vi "main(Test DQMH modules).vi"() -> ()   [LabVIEW 2018, in "Application.lvlib"] (continued)
            n1625 = Select(t="Quece timeout", s=w3888, f=w3885) -> (s? t:f=w3884:string)
            n1626 = call "string log (SubVI).vi"("Enum"=enum16{"Init", "Log", "Read"}."Log", "state Name"=w3884) -> ()  [unwired: 8 in, 2 out]
          }
          frame condition #1 {
          }
        }
        n1627 = call "progress string(SubVI).vi"("String 3"=w3850, "String in"=w3851) -> ("String out"=w3852:string)  [unwired: 9 in]
        n1628 = call "FGV Driver Data.vi"("DUT index(1-60)"=w3849) -> ("DUT SC"=w3848:bool)  [unwired: 7 in, 3 out]
        n1629 = case shown="False" w3848 {
          tunnel: [w3877 _] -> w3857
          tunnel: w3854 -> [w3876 _]
          frame False {
            w3864 = T11 {"command"="", "command data"=variant} ("element")
            w3863 = "MEAS.mux6_1"
            n1630 = To Variant(anything=T4."mux6-1_channel0" ("mux6_1(3wires)_encode")) -> (Variant=w3862:variant)
            n1631 = To Variant(anything=T4."mux6_1_channel1_3" ("mux6_1(3wires)_encode")) -> (Variant=w3874:variant)
            n1632 = To Variant(anything=T4."mux6-1_channel1_2" ("mux6_1(3wires)_encode")) -> (Variant=w3872:variant)
            n1633 = Bundle By Name(cluster=w3864, "command"=w3863, "command data"=w3872) -> (w3871:T11)
            n1634 = Bundle By Name(cluster=w3864, "command"=w3863, "command data"=w3874) -> (w3870:T11)
            n1635 = Bundle By Name(cluster=w3864, "command"=w3863, "command data"=w3862) -> ()  [unwired: 1 out]
            n1636 = Bundle By Name(cluster=w3864, "command"="MEAS.DMM dual read") -> (w3868:T11)
            n1637 = Build Array(w3871, w3870, w3868) -> (w3866:T11[])
            n1638 = Reverse 1D Array(array=w3866) -> (reversed array=w3867:T11[])
            n1639 = for {
              tunnel: [w3883] -> w3877 mode=indexing
              tunnel: w3876 -> [w3882]
              tunnel: w3867 -> [w3881] mode=indexing
              n1640 = Unbundle By Name(w3881) -> ("command"=w3880:string, "command data"=w3879:variant)
              n1641 = call "App enquece.vi"("Priority Enquece"=TRUE, "command data"=w3879, "command"=w3880, "queue in"=w3882) -> ("error out"=w3883:errorcluster)  [unwired: 6 in, 1 out]
            }
          }
          frame True {
          }
        }
        n1642 = Merge Errors(w3855, w3857) -> (w3856:errorcluster)
      }
      frame "Test DRV 8" {
        w3890 = 8  # DUT index(0-59)
        n1643 = disable-structure shown="LOGGING==TRUE" {
          disable-tunnel: w3891 -> [w3926 _]
          frame condition #0 (active) {
            n1644 = Empty String/Path?(string/path=w3926) -> (empty?=w3929:bool)
            n1645 = Select(t="Quece timeout", s=w3929, f=w3926) -> (s? t:f=w3925:string)
            n1646 = call "string log (SubVI).vi"("Enum"=enum16{"Init", "Log", "Read"}."Log", "state Name"=w3925) -> ()  [unwired: 8 in, 2 out]
          }
          frame condition #1 {
          }
        }
        n1647 = call "progress string(SubVI).vi"("String 3"=w3891, "String in"=w3892) -> ("String out"=w3893:string)  [unwired: 9 in]
        n1648 = call "FGV Driver Data.vi"("DUT index(1-60)"=w3890) -> ("DUT SC"=w3889:bool)  [unwired: 7 in, 3 out]
        n1649 = case shown="False" w3889 {
          tunnel: [w3918 _] -> w3898
          tunnel: w3895 -> [w3917 _]
          frame False {
            w3905 = T11 {"command"="", "command data"=variant} ("element")
            w3904 = "MEAS.mux6_1"
            n1650 = To Variant(anything=T4."mux6-1_channel0" ("mux6_1(3wires)_encode")) -> (Variant=w3903:variant)
            n1651 = To Variant(anything=T4."mux6_1_channel2_3" ("mux6_1(3wires)_encode")) -> (Variant=w3915:variant)
            n1652 = To Variant(anything=T4."mux6_1_channel2_2" ("mux6_1(3wires)_encode")) -> (Variant=w3913:variant)
            n1653 = Bundle By Name(cluster=w3905, "command"=w3904, "command data"=w3913) -> (w3912:T11)
            n1654 = Bundle By Name(cluster=w3905, "command"=w3904, "command data"=w3915) -> (w3911:T11)
            n1655 = Bundle By Name(cluster=w3905, "command"=w3904, "command data"=w3903) -> ()  [unwired: 1 out]
            n1656 = Bundle By Name(cluster=w3905, "command"="MEAS.DMM dual read") -> (w3909:T11)
            n1657 = Build Array(w3912, w3911, w3909) -> (w3907:T11[])
            n1658 = Reverse 1D Array(array=w3907) -> (reversed array=w3908:T11[])
            n1659 = for {
              tunnel: [w3924] -> w3918 mode=indexing
              tunnel: w3917 -> [w3923]
              tunnel: w3908 -> [w3922] mode=indexing
              n1660 = Unbundle By Name(w3922) -> ("command"=w3921:string, "command data"=w3920:variant)
              n1661 = call "App enquece.vi"("Priority Enquece"=TRUE, "command data"=w3920, "command"=w3921, "queue in"=w3923) -> ("error out"=w3924:errorcluster)  [unwired: 6 in, 1 out]
            }
          }
          frame True {
          }
        }
        n1662 = Merge Errors(w3896, w3898) -> (w3897:errorcluster)
      }
      frame "Test DRV 9" {
        w3931 = 9  # DUT index(0-59)
        n1663 = disable-structure shown="LOGGING==TRUE" {
          disable-tunnel: w3932 -> [w3967 _]
          frame condition #0 (active) {
            n1664 = Empty String/Path?(string/path=w3967) -> (empty?=w3970:bool)
            n1665 = Select(t="Quece timeout", s=w3970, f=w3967) -> (s? t:f=w3966:string)
            n1666 = call "string log (SubVI).vi"("Enum"=enum16{"Init", "Log", "Read"}."Log", "state Name"=w3966) -> ()  [unwired: 8 in, 2 out]
          }
          frame condition #1 {
          }
        }
        n1667 = call "progress string(SubVI).vi"("String 3"=w3932, "String in"=w3933) -> ("String out"=w3934:string)  [unwired: 9 in]
        n1668 = call "FGV Driver Data.vi"("DUT index(1-60)"=w3931) -> ("DUT SC"=w3930:bool)  [unwired: 7 in, 3 out]
        n1669 = case shown="False" w3930 {
          tunnel: [w3959 _] -> w3939
          tunnel: w3936 -> [w3958 _]
          frame False {
            w3946 = T11 {"command"="", "command data"=variant} ("element")
            w3945 = "MEAS.mux6_1"
            n1670 = To Variant(anything=T4."mux6-1_channel0" ("mux6_1(3wires)_encode")) -> (Variant=w3944:variant)
            n1671 = To Variant(anything=T4."mux6_1_channel3_3" ("mux6_1(3wires)_encode")) -> (Variant=w3956:variant)
            n1672 = To Variant(anything=T4."mux6_1_channel3_2" ("mux6_1(3wires)_encode")) -> (Variant=w3954:variant)
            n1673 = Bundle By Name(cluster=w3946, "command"=w3945, "command data"=w3954) -> (w3953:T11)
            n1674 = Bundle By Name(cluster=w3946, "command"=w3945, "command data"=w3956) -> (w3952:T11)
            n1675 = Bundle By Name(cluster=w3946, "command"=w3945, "command data"=w3944) -> ()  [unwired: 1 out]
            n1676 = Bundle By Name(cluster=w3946, "command"="MEAS.DMM dual read") -> (w3950:T11)
            n1677 = Build Array(w3953, w3952, w3950) -> (w3948:T11[])
            n1678 = Reverse 1D Array(array=w3948) -> (reversed array=w3949:T11[])
            n1679 = for {
              tunnel: [w3965] -> w3959 mode=indexing
              tunnel: w3958 -> [w3964]
              tunnel: w3949 -> [w3963] mode=indexing
              n1680 = Unbundle By Name(w3963) -> ("command"=w3962:string, "command data"=w3961:variant)
              n1681 = call "App enquece.vi"("Priority Enquece"=TRUE, "command data"=w3961, "command"=w3962, "queue in"=w3964) -> ("error out"=w3965:errorcluster)  [unwired: 6 in, 1 out]
            }
          }
          frame True {
          }
        }
        n1682 = Merge Errors(w3937, w3939) -> (w3938:errorcluster)
      }
      frame "Test DRV 10" {
        w3972 = 10  # DUT index(0-59)
        n1683 = disable-structure shown="LOGGING==TRUE" {
          disable-tunnel: w3973 -> [w4008 _]
          frame condition #0 (active) {
            n1684 = Empty String/Path?(string/path=w4008) -> (empty?=w4011:bool)
            n1685 = Select(t="Quece timeout", s=w4011, f=w4008) -> (s? t:f=w4007:string)
            n1686 = call "string log (SubVI).vi"("Enum"=enum16{"Init", "Log", "Read"}."Log", "state Name"=w4007) -> ()  [unwired: 8 in, 2 out]
          }
          frame condition #1 {
          }
        }
        n1687 = call "progress string(SubVI).vi"("String 3"=w3973, "String in"=w3974) -> ("String out"=w3975:string)  [unwired: 9 in]
        n1688 = call "FGV Driver Data.vi"("DUT index(1-60)"=w3972) -> ("DUT SC"=w3971:bool)  [unwired: 7 in, 3 out]
        n1689 = case shown="False" w3971 {
          tunnel: [w4000 _] -> w3980
          tunnel: w3977 -> [w3999 _]
          frame False {
            w3987 = T11 {"command"="", "command data"=variant} ("element")
            w3986 = "MEAS.mux6_1"
            n1690 = To Variant(anything=T4."mux6-1_channel0" ("mux6_1(3wires)_encode")) -> (Variant=w3985:variant)
            n1691 = To Variant(anything=T4."mux6_1_channel4_3" ("mux6_1(3wires)_encode")) -> (Variant=w3997:variant)
            n1692 = To Variant(anything=T4."mux6_1_channel4_2" ("mux6_1(3wires)_encode")) -> (Variant=w3995:variant)
            n1693 = Bundle By Name(cluster=w3987, "command"=w3986, "command data"=w3995) -> (w3994:T11)
            n1694 = Bundle By Name(cluster=w3987, "command"=w3986, "command data"=w3997) -> (w3993:T11)
            n1695 = Bundle By Name(cluster=w3987, "command"=w3986, "command data"=w3985) -> ()  [unwired: 1 out]
            n1696 = Bundle By Name(cluster=w3987, "command"="MEAS.DMM dual read") -> (w3991:T11)
            n1697 = Build Array(w3994, w3993, w3991) -> (w3989:T11[])
            n1698 = Reverse 1D Array(array=w3989) -> (reversed array=w3990:T11[])
            n1699 = for {
              tunnel: [w4006] -> w4000 mode=indexing
              tunnel: w3999 -> [w4005]
              tunnel: w3990 -> [w4004] mode=indexing
              n1700 = Unbundle By Name(w4004) -> ("command"=w4003:string, "command data"=w4002:variant)
              n1701 = call "App enquece.vi"("Priority Enquece"=TRUE, "command data"=w4002, "command"=w4003, "queue in"=w4005) -> ("error out"=w4006:errorcluster)  [unwired: 6 in, 1 out]
            }
          }
          frame True {
          }
        }
        n1702 = Merge Errors(w3978, w3980) -> (w3979:errorcluster)
      }
      frame "Test DRV 11" {
        w4013 = 11  # DUT index(0-59)
        n1703 = disable-structure shown="LOGGING==TRUE" {
          disable-tunnel: w4014 -> [w4049 _]
          frame condition #0 (active) {
            n1704 = Empty String/Path?(string/path=w4049) -> (empty?=w4052:bool)
            n1705 = Select(t="Quece timeout", s=w4052, f=w4049) -> (s? t:f=w4048:string)
            n1706 = call "string log (SubVI).vi"("Enum"=enum16{"Init", "Log", "Read"}."Log", "state Name"=w4048) -> ()  [unwired: 8 in, 2 out]
          }
          frame condition #1 {
          }
        }
        n1707 = call "progress string(SubVI).vi"("String 3"=w4014, "String in"=w4015) -> ("String out"=w4016:string)  [unwired: 9 in]
        n1708 = call "FGV Driver Data.vi"("DUT index(1-60)"=w4013) -> ("DUT SC"=w4012:bool)  [unwired: 7 in, 3 out]
        n1709 = case shown="False" w4012 {
          tunnel: [w4041 _] -> w4021
          tunnel: w4018 -> [w4040 _]
          frame False {
            w4026 = T11 {"command"="", "command data"=variant} ("element")
            w4028 = "MEAS.mux6_1"
            n1710 = To Variant(anything=T4."mux6-1_channel0" ("mux6_1(3wires)_encode")) -> (Variant=w4027:variant)
            n1711 = To Variant(anything=T4."mux6_1_channel5_3" ("mux6_1(3wires)_encode")) -> (Variant=w4038:variant)
            n1712 = To Variant(anything=T4."mux6_1_channel5_2" ("mux6_1(3wires)_encode")) -> (Variant=w4036:variant)
            n1713 = Bundle By Name(cluster=w4026, "command"=w4028, "command data"=w4036) -> (w4035:T11)
            n1714 = Bundle By Name(cluster=w4026, "command"=w4028, "command data"=w4038) -> (w4034:T11)
            n1715 = Bundle By Name(cluster=w4026, "command"=w4028, "command data"=w4027) -> ()  [unwired: 1 out]
            n1716 = Bundle By Name(cluster=w4026, "command"="MEAS.DMM dual read") -> (w4032:T11)
            n1717 = Build Array(w4035, w4034, w4032) -> (w4030:T11[])
            n1718 = Reverse 1D Array(array=w4030) -> (reversed array=w4031:T11[])
            n1719 = for {
              tunnel: [w4047] -> w4041 mode=indexing
              tunnel: w4040 -> [w4046]
              tunnel: w4031 -> [w4045] mode=indexing
              n1720 = Unbundle By Name(w4045) -> ("command"=w4044:string, "command data"=w4043:variant)
              n1721 = call "App enquece.vi"("Priority Enquece"=TRUE, "command data"=w4043, "command"=w4044, "queue in"=w4046) -> ("error out"=w4047:errorcluster)  [unwired: 6 in, 1 out]
            }
          }
          frame True {
          }
        }
        n1722 = Merge Errors(w4019, w4021) -> (w4020:errorcluster)
      }
      frame "Test DRV 12" {
        w4054 = 12  # DUT index(0-59)
        n1723 = disable-structure shown="LOGGING==TRUE" {
          disable-tunnel: w4055 -> [w4090 _]
          frame condition #0 (active) {
            n1724 = Empty String/Path?(string/path=w4090) -> (empty?=w4093:bool)
            n1725 = Select(t="Quece timeout", s=w4093, f=w4090) -> (s? t:f=w4089:string)
            n1726 = call "string log (SubVI).vi"("Enum"=enum16{"Init", "Log", "Read"}."Log", "state Name"=w4089) -> ()  [unwired: 8 in, 2 out]
          }
          frame condition #1 {
          }
        }
        n1727 = call "progress string(SubVI).vi"("String 3"=w4055, "String in"=w4056) -> ("String out"=w4057:string)  [unwired: 9 in]
        n1728 = call "FGV Driver Data.vi"("DUT index(1-60)"=w4054) -> ("DUT SC"=w4053:bool)  [unwired: 7 in, 3 out]
        n1729 = case shown="False" w4053 {
          tunnel: [w4082 _] -> w4062
          tunnel: w4059 -> [w4081 _]
          frame False {
            w4069 = T11 {"command"="", "command data"=variant} ("element")
            w4068 = "MEAS.mux6_1"
            n1730 = To Variant(anything=T4."mux6-1_channel0" ("mux6_1(3wires)_encode")) -> (Variant=w4067:variant)
            n1731 = To Variant(anything=T4."mux6_1_channel6_3" ("mux6_1(3wires)_encode")) -> (Variant=w4079:variant)
            n1732 = To Variant(anything=T4."mux6_1_channel6_2" ("mux6_1(3wires)_encode")) -> (Variant=w4077:variant)
            n1733 = Bundle By Name(cluster=w4069, "command"=w4068, "command data"=w4077) -> (w4076:T11)
            n1734 = Bundle By Name(cluster=w4069, "command"=w4068, "command data"=w4079) -> (w4075:T11)
            n1735 = Bundle By Name(cluster=w4069, "command"=w4068, "command data"=w4067) -> ()  [unwired: 1 out]
            n1736 = Bundle By Name(cluster=w4069, "command"="MEAS.DMM dual read") -> (w4073:T11)
            n1737 = Build Array(w4076, w4075, w4073) -> (w4071:T11[])
            n1738 = Reverse 1D Array(array=w4071) -> (reversed array=w4072:T11[])
            n1739 = for {
              tunnel: [w4088] -> w4082 mode=indexing
              tunnel: w4081 -> [w4087]
              tunnel: w4072 -> [w4086] mode=indexing
              n1740 = Unbundle By Name(w4086) -> ("command"=w4085:string, "command data"=w4084:variant)
              n1741 = call "App enquece.vi"("Priority Enquece"=TRUE, "command data"=w4084, "command"=w4085, "queue in"=w4087) -> ("error out"=w4088:errorcluster)  [unwired: 6 in, 1 out]
            }
          }
          frame True {
          }
        }
        n1742 = Merge Errors(w4060, w4062) -> (w4061:errorcluster)
      }
      frame "Test DRV 13" {
        w4095 = 13  # DUT index(0-59)
        n1743 = disable-structure shown="LOGGING==TRUE" {
          disable-tunnel: w4096 -> [w4131 _]
          frame condition #0 (active) {
            n1744 = Empty String/Path?(string/path=w4131) -> (empty?=w4134:bool)
            n1745 = Select(t="Quece timeout", s=w4134, f=w4131) -> (s? t:f=w4130:string)
            n1746 = call "string log (SubVI).vi"("Enum"=enum16{"Init", "Log", "Read"}."Log", "state Name"=w4130) -> ()  [unwired: 8 in, 2 out]
          }
          frame condition #1 {
          }
        }
        n1747 = call "progress string(SubVI).vi"("String 3"=w4096, "String in"=w4097) -> ("String out"=w4098:string)  [unwired: 9 in]
        n1748 = call "FGV Driver Data.vi"("DUT index(1-60)"=w4095) -> ("DUT SC"=w4094:bool)  [unwired: 7 in, 3 out]
        n1749 = case shown="False" w4094 {
          tunnel: [w4123 _] -> w4103
          tunnel: w4100 -> [w4122 _]
          frame False {
            w4110 = T11 {"command"="", "command data"=variant} ("element")
            w4109 = "MEAS.mux6_1"
            n1750 = To Variant(anything=T4."mux6-1_channel0" ("mux6_1(3wires)_encode")) -> (Variant=w4108:variant)
            n1751 = To Variant(anything=T4."mux6_1_channel1_3" ("mux6_1(3wires)_encode")) -> (Variant=w4120:variant)
            n1752 = To Variant(anything=T4."mux6-1_channel1_2" ("mux6_1(3wires)_encode")) -> (Variant=w4118:variant)
            n1753 = Bundle By Name(cluster=w4110, "command"=w4109, "command data"=w4118) -> (w4117:T11)
            n1754 = Bundle By Name(cluster=w4110, "command"=w4109, "command data"=w4120) -> (w4116:T11)
            n1755 = Bundle By Name(cluster=w4110, "command"=w4109, "command data"=w4108) -> ()  [unwired: 1 out]
            n1756 = Bundle By Name(cluster=w4110, "command"="MEAS.DMM dual read") -> (w4114:T11)
            n1757 = Build Array(w4117, w4116, w4114) -> (w4112:T11[])
            n1758 = Reverse 1D Array(array=w4112) -> (reversed array=w4113:T11[])
            n1759 = for {
              tunnel: [w4129] -> w4123 mode=indexing
              tunnel: w4122 -> [w4128]
              tunnel: w4113 -> [w4127] mode=indexing
              n1760 = Unbundle By Name(w4127) -> ("command"=w4126:string, "command data"=w4125:variant)
              n1761 = call "App enquece.vi"("Priority Enquece"=TRUE, "command data"=w4125, "command"=w4126, "queue in"=w4128) -> ("error out"=w4129:errorcluster)  [unwired: 6 in, 1 out]
            }
          }
          frame True {
          }
        }
        n1762 = Merge Errors(w4101, w4103) -> (w4102:errorcluster)
      }
      frame "Test DRV 14" {
        w4136 = 14  # DUT index(0-59)
        n1763 = disable-structure shown="LOGGING==TRUE" {
          disable-tunnel: w4137 -> [w4172 _]
          frame condition #0 (active) {
            n1764 = Empty String/Path?(string/path=w4172) -> (empty?=w4175:bool)
            n1765 = Select(t="Quece timeout", s=w4175, f=w4172) -> (s? t:f=w4171:string)
            n1766 = call "string log (SubVI).vi"("Enum"=enum16{"Init", "Log", "Read"}."Log", "state Name"=w4171) -> ()  [unwired: 8 in, 2 out]
          }
          frame condition #1 {
          }
        }
        n1767 = call "progress string(SubVI).vi"("String 3"=w4137, "String in"=w4138) -> ("String out"=w4139:string)  [unwired: 9 in]
        n1768 = call "FGV Driver Data.vi"("DUT index(1-60)"=w4136) -> ("DUT SC"=w4135:bool)  [unwired: 7 in, 3 out]
        n1769 = case shown="False" w4135 {
          tunnel: [w4164 _] -> w4144
          tunnel: w4141 -> [w4163 _]
          frame False {
            w4151 = T11 {"command"="", "command data"=variant} ("element")
            w4150 = "MEAS.mux6_1"
            n1770 = To Variant(anything=T4."mux6_1_channel2_3" ("mux6_1(3wires)_encode")) -> (Variant=w4161:variant)
            n1771 = To Variant(anything=T4."mux6-1_channel0" ("mux6_1(3wires)_encode")) -> (Variant=w4149:variant)
            n1772 = To Variant(anything=T4."mux6_1_channel2_2" ("mux6_1(3wires)_encode")) -> (Variant=w4159:variant)
            n1773 = Bundle By Name(cluster=w4151, "command"=w4150, "command data"=w4159) -> (w4158:T11)
            n1774 = Bundle By Name(cluster=w4151, "command"=w4150, "command data"=w4161) -> (w4157:T11)
            n1775 = Bundle By Name(cluster=w4151, "command"=w4150, "command data"=w4149) -> ()  [unwired: 1 out]
            n1776 = Bundle By Name(cluster=w4151, "command"="MEAS.DMM dual read") -> (w4155:T11)
            n1777 = Build Array(w4158, w4157, w4155) -> (w4153:T11[])
            n1778 = Reverse 1D Array(array=w4153) -> (reversed array=w4154:T11[])
            n1779 = for {
              tunnel: [w4170] -> w4164 mode=indexing
              tunnel: w4163 -> [w4169]
              tunnel: w4154 -> [w4168] mode=indexing
              n1780 = Unbundle By Name(w4168) -> ("command"=w4167:string, "command data"=w4166:variant)
              n1781 = call "App enquece.vi"("Priority Enquece"=TRUE, "command data"=w4166, "command"=w4167, "queue in"=w4169) -> ("error out"=w4170:errorcluster)  [unwired: 6 in, 1 out]
            }
          }
          frame True {
          }
        }
        n1782 = Merge Errors(w4142, w4144) -> (w4143:errorcluster)
      }
      frame "Test DRV 15" {
        w4177 = 15  # DUT index(0-59)
        n1783 = disable-structure shown="LOGGING==TRUE" {
          disable-tunnel: w4178 -> [w4213 _]
          frame condition #0 (active) {
            n1784 = Empty String/Path?(string/path=w4213) -> (empty?=w4216:bool)
            n1785 = Select(t="Quece timeout", s=w4216, f=w4213) -> (s? t:f=w4212:string)
            n1786 = call "string log (SubVI).vi"("Enum"=enum16{"Init", "Log", "Read"}."Log", "state Name"=w4212) -> ()  [unwired: 8 in, 2 out]
          }
          frame condition #1 {
          }
        }
        n1787 = call "progress string(SubVI).vi"("String 3"=w4178, "String in"=w4179) -> ("String out"=w4180:string)  [unwired: 9 in]
        n1788 = call "FGV Driver Data.vi"("DUT index(1-60)"=w4177) -> ("DUT SC"=w4176:bool)  [unwired: 7 in, 3 out]
        n1789 = case shown="False" w4176 {
          tunnel: [w4205 _] -> w4185
          tunnel: w4182 -> [w4204 _]
          frame False {
            w4192 = T11 {"command"="", "command data"=variant} ("element")
            w4191 = "MEAS.mux6_1"
            n1790 = To Variant(anything=T4."mux6-1_channel0" ("mux6_1(3wires)_encode")) -> (Variant=w4190:variant)
            n1791 = To Variant(anything=T4."mux6_1_channel3_3" ("mux6_1(3wires)_encode")) -> (Variant=w4202:variant)
            n1792 = To Variant(anything=T4."mux6_1_channel3_2" ("mux6_1(3wires)_encode")) -> (Variant=w4200:variant)
            n1793 = Bundle By Name(cluster=w4192, "command"=w4191, "command data"=w4200) -> (w4199:T11)
            n1794 = Bundle By Name(cluster=w4192, "command"=w4191, "command data"=w4202) -> (w4198:T11)
            n1795 = Bundle By Name(cluster=w4192, "command"=w4191, "command data"=w4190) -> ()  [unwired: 1 out]
            n1796 = Bundle By Name(cluster=w4192, "command"="MEAS.DMM dual read") -> (w4196:T11)
            n1797 = Build Array(w4199, w4198, w4196) -> (w4194:T11[])
            n1798 = Reverse 1D Array(array=w4194) -> (reversed array=w4195:T11[])
            n1799 = for {
              tunnel: [w4211] -> w4205 mode=indexing
              tunnel: w4204 -> [w4210]
              tunnel: w4195 -> [w4209] mode=indexing
              n1800 = Unbundle By Name(w4209) -> ("command"=w4208:string, "command data"=w4207:variant)
              n1801 = call "App enquece.vi"("Priority Enquece"=TRUE, "command data"=w4207, "command"=w4208, "queue in"=w4210) -> ("error out"=w4211:errorcluster)  [unwired: 6 in, 1 out]
            }
          }
          frame True {
          }
        }
        n1802 = Merge Errors(w4183, w4185) -> (w4184:errorcluster)
      }
      frame "Test DRV 16" {
        w4218 = 16  # DUT index(0-59)
        n1803 = disable-structure shown="LOGGING==TRUE" {
          disable-tunnel: w4219 -> [w4254 _]
          frame condition #0 (active) {
            n1804 = Empty String/Path?(string/path=w4254) -> (empty?=w4257:bool)
            n1805 = Select(t="Quece timeout", s=w4257, f=w4254) -> (s? t:f=w4253:string)
            n1806 = call "string log (SubVI).vi"("Enum"=enum16{"Init", "Log", "Read"}."Log", "state Name"=w4253) -> ()  [unwired: 8 in, 2 out]
          }
          frame condition #1 {
          }
        }
        n1807 = call "progress string(SubVI).vi"("String 3"=w4219, "String in"=w4220) -> ("String out"=w4221:string)  [unwired: 9 in]
        n1808 = call "FGV Driver Data.vi"("DUT index(1-60)"=w4218) -> ("DUT SC"=w4217:bool)  [unwired: 7 in, 3 out]
        n1809 = case shown="False" w4217 {
          tunnel: [w4246 _] -> w4226
          tunnel: w4223 -> [w4245 _]
          frame False {
            w4233 = T11 {"command"="", "command data"=variant} ("element")
            w4232 = "MEAS.mux6_1"
            n1810 = To Variant(anything=T4."mux6-1_channel0" ("mux6_1(3wires)_encode")) -> (Variant=w4231:variant)
            n1811 = To Variant(anything=T4."mux6_1_channel4_3" ("mux6_1(3wires)_encode")) -> (Variant=w4243:variant)
            n1812 = To Variant(anything=T4."mux6_1_channel4_2" ("mux6_1(3wires)_encode")) -> (Variant=w4241:variant)
            n1813 = Bundle By Name(cluster=w4233, "command"=w4232, "command data"=w4241) -> (w4240:T11)
            n1814 = Bundle By Name(cluster=w4233, "command"=w4232, "command data"=w4243) -> (w4239:T11)
            n1815 = Bundle By Name(cluster=w4233, "command"=w4232, "command data"=w4231) -> ()  [unwired: 1 out]
            n1816 = Bundle By Name(cluster=w4233, "command"="MEAS.DMM dual read") -> (w4237:T11)
            n1817 = Build Array(w4240, w4239, w4237) -> (w4235:T11[])
            n1818 = Reverse 1D Array(array=w4235) -> (reversed array=w4236:T11[])
            n1819 = for {
              tunnel: [w4252] -> w4246 mode=indexing
              tunnel: w4245 -> [w4251]
              tunnel: w4236 -> [w4250] mode=indexing
              n1820 = Unbundle By Name(w4250) -> ("command"=w4249:string, "command data"=w4248:variant)
              n1821 = call "App enquece.vi"("Priority Enquece"=TRUE, "command data"=w4248, "command"=w4249, "queue in"=w4251) -> ("error out"=w4252:errorcluster)  [unwired: 6 in, 1 out]
            }
          }
          frame True {
          }
        }
        n1822 = Merge Errors(w4224, w4226) -> (w4225:errorcluster)
      }
      frame "Test DRV 17" {
        w4258 = 17  # DUT index(0-59)
        n1823 = disable-structure shown="LOGGING==TRUE" {
          disable-tunnel: w4260 -> [w4295 _]
          frame condition #0 (active) {
            n1824 = Empty String/Path?(string/path=w4295) -> (empty?=w4298:bool)
            n1825 = Select(t="Quece timeout", s=w4298, f=w4295) -> (s? t:f=w4294:string)
            n1826 = call "string log (SubVI).vi"("Enum"=enum16{"Init", "Log", "Read"}."Log", "state Name"=w4294) -> ()  [unwired: 8 in, 2 out]
          }
          frame condition #1 {
          }
        }
        n1827 = call "progress string(SubVI).vi"("String 3"=w4260, "String in"=w4261) -> ("String out"=w4262:string)  [unwired: 9 in]
        n1828 = call "FGV Driver Data.vi"("DUT index(1-60)"=w4258) -> ("DUT SC"=w4259:bool)  [unwired: 7 in, 3 out]
        n1829 = case shown="False" w4259 {
          tunnel: [w4287 _] -> w4267
          tunnel: w4264 -> [w4286 _]
          frame False {
            w4274 = T11 {"command"="", "command data"=variant} ("element")
            w4273 = "MEAS.mux6_1"
            n1830 = To Variant(anything=T4."mux6-1_channel0" ("mux6_1(3wires)_encode")) -> (Variant=w4272:variant)
            n1831 = To Variant(anything=T4."mux6_1_channel5_3" ("mux6_1(3wires)_encode")) -> (Variant=w4284:variant)
            n1832 = To Variant(anything=T4."mux6_1_channel5_2" ("mux6_1(3wires)_encode")) -> (Variant=w4282:variant)
            n1833 = Bundle By Name(cluster=w4274, "command"=w4273, "command data"=w4282) -> (w4281:T11)
            n1834 = Bundle By Name(cluster=w4274, "command"=w4273, "command data"=w4284) -> (w4280:T11)
            n1835 = Bundle By Name(cluster=w4274, "command"=w4273, "command data"=w4272) -> ()  [unwired: 1 out]
            n1836 = Bundle By Name(cluster=w4274, "command"="MEAS.DMM dual read") -> (w4278:T11)
            n1837 = Build Array(w4281, w4280, w4278) -> (w4276:T11[])
            n1838 = Reverse 1D Array(array=w4276) -> (reversed array=w4277:T11[])
            n1839 = for {
              tunnel: [w4293] -> w4287 mode=indexing
              tunnel: w4286 -> [w4292]
              tunnel: w4277 -> [w4291] mode=indexing
              n1840 = Unbundle By Name(w4291) -> ("command"=w4290:string, "command data"=w4289:variant)
              n1841 = call "App enquece.vi"("Priority Enquece"=TRUE, "command data"=w4289, "command"=w4290, "queue in"=w4292) -> ("error out"=w4293:errorcluster)  [unwired: 6 in, 1 out]
            }
          }
          frame True {
          }
        }
        n1842 = Merge Errors(w4265, w4267) -> (w4266:errorcluster)
      }
      frame "Test DRV 18" {
        w4302 = 18  # DUT index(0-59)
        n1843 = disable-structure shown="LOGGING==TRUE" {
          disable-tunnel: w4299 -> [w4336 _]
          frame condition #0 (active) {
            n1844 = Empty String/Path?(string/path=w4336) -> (empty?=w4339:bool)
            n1845 = Select(t="Quece timeout", s=w4339, f=w4336) -> (s? t:f=w4335:string)
            n1846 = call "string log (SubVI).vi"("Enum"=enum16{"Init", "Log", "Read"}."Log", "state Name"=w4335) -> ()  [unwired: 8 in, 2 out]
          }
          frame condition #1 {
          }
        }
        n1847 = call "progress string(SubVI).vi"("String 3"=w4299, "String in"=w4300) -> ("String out"=w4301:string)  [unwired: 9 in]
        n1848 = call "FGV Driver Data.vi"("DUT index(1-60)"=w4302) -> ("DUT SC"=w4303:bool)  [unwired: 7 in, 3 out]
        n1849 = case shown="False" w4303 {
          tunnel: [w4328 _] -> w4308
          tunnel: w4305 -> [w4327 _]
          frame False {
            w4315 = T11 {"command"="", "command data"=variant} ("element")
            w4314 = "MEAS.mux6_1"
            n1850 = To Variant(anything=T4."mux6-1_channel0" ("mux6_1(3wires)_encode")) -> (Variant=w4313:variant)
            n1851 = To Variant(anything=T4."mux6_1_channel6_3" ("mux6_1(3wires)_encode")) -> (Variant=w4325:variant)
            n1852 = To Variant(anything=T4."mux6_1_channel6_2" ("mux6_1(3wires)_encode")) -> (Variant=w4323:variant)
            n1853 = Bundle By Name(cluster=w4315, "command"=w4314, "command data"=w4323) -> (w4322:T11)
            n1854 = Bundle By Name(cluster=w4315, "command"=w4314, "command data"=w4325) -> (w4321:T11)
            n1855 = Bundle By Name(cluster=w4315, "command"=w4314, "command data"=w4313) -> ()  [unwired: 1 out]
            n1856 = Bundle By Name(cluster=w4315, "command"="MEAS.DMM dual read") -> (w4319:T11)
            n1857 = Build Array(w4322, w4321, w4319) -> (w4317:T11[])
            n1858 = Reverse 1D Array(array=w4317) -> (reversed array=w4318:T11[])
            n1859 = for {
              tunnel: [w4334] -> w4328 mode=indexing
              tunnel: w4327 -> [w4333]
              tunnel: w4318 -> [w4332] mode=indexing
              n1860 = Unbundle By Name(w4332) -> ("command"=w4331:string, "command data"=w4330:variant)
              n1861 = call "App enquece.vi"("Priority Enquece"=TRUE, "command data"=w4330, "command"=w4331, "queue in"=w4333) -> ("error out"=w4334:errorcluster)  [unwired: 6 in, 1 out]
            }
          }
          frame True {
          }
        }
        n1862 = Merge Errors(w4306, w4308) -> (w4307:errorcluster)
      }
      frame "Test DRV 19" {
        w4341 = 19  # DUT index(0-59)
        n1863 = disable-structure shown="LOGGING==TRUE" {
          disable-tunnel: w4342 -> [w4377 _]
          frame condition #0 (active) {
            n1864 = Empty String/Path?(string/path=w4377) -> (empty?=w4380:bool)
            n1865 = Select(t="Quece timeout", s=w4380, f=w4377) -> (s? t:f=w4376:string)
            n1866 = call "string log (SubVI).vi"("Enum"=enum16{"Init", "Log", "Read"}."Log", "state Name"=w4376) -> ()  [unwired: 8 in, 2 out]
          }
          frame condition #1 {
          }
        }
        n1867 = call "progress string(SubVI).vi"("String 3"=w4342, "String in"=w4343) -> ("String out"=w4344:string)  [unwired: 9 in]
        n1868 = call "FGV Driver Data.vi"("DUT index(1-60)"=w4341) -> ("DUT SC"=w4340:bool)  [unwired: 7 in, 3 out]
        n1869 = case shown="False" w4340 {
          tunnel: [w4369 _] -> w4349
          tunnel: w4346 -> [w4368 _]
          frame False {
            w4356 = T11 {"command"="", "command data"=variant} ("element")
            w4355 = "MEAS.mux6_1"
            n1870 = To Variant(anything=T4."mux6-1_channel0" ("mux6_1(3wires)_encode")) -> (Variant=w4354:variant)
            n1871 = To Variant(anything=T4."mux6_1_channel1_3" ("mux6_1(3wires)_encode")) -> (Variant=w4366:variant)
            n1872 = To Variant(anything=T4."mux6-1_channel1_2" ("mux6_1(3wires)_encode")) -> (Variant=w4364:variant)
            n1873 = Bundle By Name(cluster=w4356, "command"=w4355, "command data"=w4364) -> (w4363:T11)
            n1874 = Bundle By Name(cluster=w4356, "command"=w4355, "command data"=w4366) -> (w4362:T11)
            n1875 = Bundle By Name(cluster=w4356, "command"=w4355, "command data"=w4354) -> ()  [unwired: 1 out]
            n1876 = Bundle By Name(cluster=w4356, "command"="MEAS.DMM dual read") -> (w4360:T11)
            n1877 = Build Array(w4363, w4362, w4360) -> (w4358:T11[])
            n1878 = Reverse 1D Array(array=w4358) -> (reversed array=w4359:T11[])
            n1879 = for {
              tunnel: [w4375] -> w4369 mode=indexing
              tunnel: w4368 -> [w4374]
              tunnel: w4359 -> [w4373] mode=indexing
              n1880 = Unbundle By Name(w4373) -> ("command"=w4372:string, "command data"=w4371:variant)
              n1881 = call "App enquece.vi"("Priority Enquece"=TRUE, "command data"=w4371, "command"=w4372, "queue in"=w4374) -> ("error out"=w4375:errorcluster)  [unwired: 6 in, 1 out]
            }
          }
          frame True {
          }
        }
        n1882 = Merge Errors(w4347, w4349) -> (w4348:errorcluster)
      }
      frame "Test DRV 20" {
        w4382 = 20  # DUT index(0-59)
        n1883 = disable-structure shown="LOGGING==TRUE" {
          disable-tunnel: w4383 -> [w4418 _]
          frame condition #0 (active) {
            n1884 = Empty String/Path?(string/path=w4418) -> (empty?=w4421:bool)
            n1885 = Select(t="Quece timeout", s=w4421, f=w4418) -> (s? t:f=w4417:string)
            n1886 = call "string log (SubVI).vi"("Enum"=enum16{"Init", "Log", "Read"}."Log", "state Name"=w4417) -> ()  [unwired: 8 in, 2 out]
          }
          frame condition #1 {
          }
        }
        n1887 = call "progress string(SubVI).vi"("String 3"=w4383, "String in"=w4384) -> ("String out"=w4385:string)  [unwired: 9 in]
        n1888 = call "FGV Driver Data.vi"("DUT index(1-60)"=w4382) -> ("DUT SC"=w4381:bool)  [unwired: 7 in, 3 out]
        n1889 = case shown="False" w4381 {
          tunnel: [w4410 _] -> w4390
          tunnel: w4387 -> [w4409 _]
          frame False {
            w4397 = T11 {"command"="", "command data"=variant} ("element")
            w4396 = "MEAS.mux6_1"
            n1890 = To Variant(anything=T4."mux6-1_channel0" ("mux6_1(3wires)_encode")) -> (Variant=w4395:variant)
            n1891 = To Variant(anything=T4."mux6_1_channel2_3" ("mux6_1(3wires)_encode")) -> (Variant=w4407:variant)
            n1892 = To Variant(anything=T4."mux6_1_channel2_2" ("mux6_1(3wires)_encode")) -> (Variant=w4405:variant)
            n1893 = Bundle By Name(cluster=w4397, "command"=w4396, "command data"=w4405) -> (w4404:T11)
            n1894 = Bundle By Name(cluster=w4397, "command"=w4396, "command data"=w4407) -> (w4403:T11)
            n1895 = Bundle By Name(cluster=w4397, "command"=w4396, "command data"=w4395) -> ()  [unwired: 1 out]
            n1896 = Bundle By Name(cluster=w4397, "command"="MEAS.DMM dual read") -> (w4401:T11)
            n1897 = Build Array(w4404, w4403, w4401) -> (w4399:T11[])
            n1898 = Reverse 1D Array(array=w4399) -> (reversed array=w4400:T11[])
            n1899 = for {
              tunnel: [w4416] -> w4410 mode=indexing
              tunnel: w4409 -> [w4415]
              tunnel: w4400 -> [w4414] mode=indexing
              n1900 = Unbundle By Name(w4414) -> ("command"=w4413:string, "command data"=w4412:variant)
              n1901 = call "App enquece.vi"("Priority Enquece"=TRUE, "command data"=w4412, "command"=w4413, "queue in"=w4415) -> ("error out"=w4416:errorcluster)  [unwired: 6 in, 1 out]
            }
          }
          frame True {
          }
        }
        n1902 = Merge Errors(w4388, w4390) -> (w4389:errorcluster)
      }
      frame "Test DRV 21" {
        w4423 = 21  # DUT index(0-59)
        n1903 = disable-structure shown="LOGGING==TRUE" {
          disable-tunnel: w4424 -> [w4459 _]
          frame condition #0 (active) {
            n1904 = Empty String/Path?(string/path=w4459) -> (empty?=w4462:bool)
            n1905 = Select(t="Quece timeout", s=w4462, f=w4459) -> (s? t:f=w4458:string)
            n1906 = call "string log (SubVI).vi"("Enum"=enum16{"Init", "Log", "Read"}."Log", "state Name"=w4458) -> ()  [unwired: 8 in, 2 out]
          }
          frame condition #1 {
          }
        }
        n1907 = call "progress string(SubVI).vi"("String 3"=w4424, "String in"=w4425) -> ("String out"=w4426:string)  [unwired: 9 in]
        n1908 = call "FGV Driver Data.vi"("DUT index(1-60)"=w4423) -> ("DUT SC"=w4422:bool)  [unwired: 7 in, 3 out]
        n1909 = case shown="False" w4422 {
          tunnel: [w4451 _] -> w4431
          tunnel: w4428 -> [w4450 _]
          frame False {
            w4438 = T11 {"command"="", "command data"=variant} ("element")
            w4437 = "MEAS.mux6_1"
            n1910 = To Variant(anything=T4."mux6-1_channel0" ("mux6_1(3wires)_encode")) -> (Variant=w4436:variant)
            n1911 = To Variant(anything=T4."mux6_1_channel3_3" ("mux6_1(3wires)_encode")) -> (Variant=w4448:variant)
            n1912 = To Variant(anything=T4."mux6_1_channel3_2" ("mux6_1(3wires)_encode")) -> (Variant=w4446:variant)
            n1913 = Bundle By Name(cluster=w4438, "command"=w4437, "command data"=w4446) -> (w4445:T11)
            n1914 = Bundle By Name(cluster=w4438, "command"=w4437, "command data"=w4448) -> (w4444:T11)
            n1915 = Bundle By Name(cluster=w4438, "command"=w4437, "command data"=w4436) -> ()  [unwired: 1 out]
            n1916 = Bundle By Name(cluster=w4438, "command"="MEAS.DMM dual read") -> (w4442:T11)
            n1917 = Build Array(w4445, w4444, w4442) -> (w4440:T11[])
            n1918 = Reverse 1D Array(array=w4440) -> (reversed array=w4441:T11[])
            n1919 = for {
              tunnel: [w4457] -> w4451 mode=indexing
              tunnel: w4450 -> [w4456]
              tunnel: w4441 -> [w4455] mode=indexing
              n1920 = Unbundle By Name(w4455) -> ("command"=w4454:string, "command data"=w4453:variant)
              n1921 = call "App enquece.vi"("Priority Enquece"=TRUE, "command data"=w4453, "command"=w4454, "queue in"=w4456) -> ("error out"=w4457:errorcluster)  [unwired: 6 in, 1 out]
            }
          }
          frame True {
          }
        }
        n1922 = Merge Errors(w4429, w4431) -> (w4430:errorcluster)
      }
      frame "Test DRV 22" {
        w4464 = 22  # DUT index(0-59)
        n1923 = disable-structure shown="LOGGING==TRUE" {
          disable-tunnel: w4465 -> [w4500 _]
          frame condition #0 (active) {
            n1924 = Empty String/Path?(string/path=w4500) -> (empty?=w4503:bool)
            n1925 = Select(t="Quece timeout", s=w4503, f=w4500) -> (s? t:f=w4499:string)
            n1926 = call "string log (SubVI).vi"("Enum"=enum16{"Init", "Log", "Read"}."Log", "state Name"=w4499) -> ()  [unwired: 8 in, 2 out]
          }
          frame condition #1 {
          }
        }
        n1927 = call "progress string(SubVI).vi"("String 3"=w4465, "String in"=w4466) -> ("String out"=w4467:string)  [unwired: 9 in]
        n1928 = call "FGV Driver Data.vi"("DUT index(1-60)"=w4464) -> ("DUT SC"=w4463:bool)  [unwired: 7 in, 3 out]
        n1929 = case shown="False" w4463 {
          tunnel: [w4492 _] -> w4472
          tunnel: w4469 -> [w4491 _]
          frame False {
            w4479 = T11 {"command"="", "command data"=variant} ("element")
            w4478 = "MEAS.mux6_1"
            n1930 = To Variant(anything=T4."mux6-1_channel0" ("mux6_1(3wires)_encode")) -> (Variant=w4477:variant)
            n1931 = To Variant(anything=T4."mux6_1_channel4_3" ("mux6_1(3wires)_encode")) -> (Variant=w4489:variant)
            n1932 = To Variant(anything=T4."mux6_1_channel4_2" ("mux6_1(3wires)_encode")) -> (Variant=w4487:variant)
            n1933 = Bundle By Name(cluster=w4479, "command"=w4478, "command data"=w4487) -> (w4486:T11)
            n1934 = Bundle By Name(cluster=w4479, "command"=w4478, "command data"=w4489) -> (w4485:T11)
            n1935 = Bundle By Name(cluster=w4479, "command"=w4478, "command data"=w4477) -> ()  [unwired: 1 out]
            n1936 = Bundle By Name(cluster=w4479, "command"="MEAS.DMM dual read") -> (w4483:T11)
            n1937 = Build Array(w4486, w4485, w4483) -> (w4481:T11[])
            n1938 = Reverse 1D Array(array=w4481) -> (reversed array=w4482:T11[])
            n1939 = for {
              tunnel: [w4498] -> w4492 mode=indexing
              tunnel: w4491 -> [w4497]
              tunnel: w4482 -> [w4496] mode=indexing
              n1940 = Unbundle By Name(w4496) -> ("command"=w4495:string, "command data"=w4494:variant)
              n1941 = call "App enquece.vi"("Priority Enquece"=TRUE, "command data"=w4494, "command"=w4495, "queue in"=w4497) -> ("error out"=w4498:errorcluster)  [unwired: 6 in, 1 out]
            }
          }
          frame True {
          }
        }
        n1942 = Merge Errors(w4470, w4472) -> (w4471:errorcluster)
      }
      frame "Test DRV 23" {
        w4505 = 23  # DUT index(0-59)
        n1943 = disable-structure shown="LOGGING==TRUE" {
          disable-tunnel: w4506 -> [w4541 _]
          frame condition #0 (active) {
            n1944 = Empty String/Path?(string/path=w4541) -> (empty?=w4544:bool)
            n1945 = Select(t="Quece timeout", s=w4544, f=w4541) -> (s? t:f=w4540:string)
            n1946 = call "string log (SubVI).vi"("Enum"=enum16{"Init", "Log", "Read"}."Log", "state Name"=w4540) -> ()  [unwired: 8 in, 2 out]
          }
          frame condition #1 {
          }
        }
        n1947 = call "progress string(SubVI).vi"("String 3"=w4506, "String in"=w4507) -> ("String out"=w4508:string)  [unwired: 9 in]
        n1948 = call "FGV Driver Data.vi"("DUT index(1-60)"=w4505) -> ("DUT SC"=w4504:bool)  [unwired: 7 in, 3 out]
        n1949 = case shown="False" w4504 {
          tunnel: [w4533 _] -> w4513
          tunnel: w4510 -> [w4532 _]
          frame False {
            w4520 = T11 {"command"="", "command data"=variant} ("element")
            w4519 = "MEAS.mux6_1"
            n1950 = To Variant(anything=T4."mux6-1_channel0" ("mux6_1(3wires)_encode")) -> (Variant=w4518:variant)
            n1951 = To Variant(anything=T4."mux6_1_channel5_3" ("mux6_1(3wires)_encode")) -> (Variant=w4530:variant)
            n1952 = To Variant(anything=T4."mux6_1_channel5_2" ("mux6_1(3wires)_encode")) -> (Variant=w4528:variant)
            n1953 = Bundle By Name(cluster=w4520, "command"=w4519, "command data"=w4528) -> (w4527:T11)
            n1954 = Bundle By Name(cluster=w4520, "command"=w4519, "command data"=w4530) -> (w4526:T11)
            n1955 = Bundle By Name(cluster=w4520, "command"=w4519, "command data"=w4518) -> ()  [unwired: 1 out]
            n1956 = Bundle By Name(cluster=w4520, "command"="MEAS.DMM dual read") -> (w4524:T11)
            n1957 = Build Array(w4527, w4526, w4524) -> (w4522:T11[])
            n1958 = Reverse 1D Array(array=w4522) -> (reversed array=w4523:T11[])
            n1959 = for {
              tunnel: [w4539] -> w4533 mode=indexing
              tunnel: w4532 -> [w4538]
              tunnel: w4523 -> [w4537] mode=indexing
              n1960 = Unbundle By Name(w4537) -> ("command"=w4536:string, "command data"=w4535:variant)
              n1961 = call "App enquece.vi"("Priority Enquece"=TRUE, "command data"=w4535, "command"=w4536, "queue in"=w4538) -> ("error out"=w4539:errorcluster)  [unwired: 6 in, 1 out]
            }
          }
          frame True {
          }
        }
        n1962 = Merge Errors(w4511, w4513) -> (w4512:errorcluster)
      }
      frame "Test DRV 24" {
        w4546 = 24  # DUT index(0-59)
        n1963 = disable-structure shown="LOGGING==TRUE" {
          disable-tunnel: w4547 -> [w4582 _]
          frame condition #0 (active) {
            n1964 = Empty String/Path?(string/path=w4582) -> (empty?=w4585:bool)
            n1965 = Select(t="Quece timeout", s=w4585, f=w4582) -> (s? t:f=w4581:string)
            n1966 = call "string log (SubVI).vi"("Enum"=enum16{"Init", "Log", "Read"}."Log", "state Name"=w4581) -> ()  [unwired: 8 in, 2 out]
          }
          frame condition #1 {
          }
        }
        n1967 = call "progress string(SubVI).vi"("String 3"=w4547, "String in"=w4548) -> ("String out"=w4549:string)  [unwired: 9 in]
        n1968 = call "FGV Driver Data.vi"("DUT index(1-60)"=w4546) -> ("DUT SC"=w4545:bool)  [unwired: 7 in, 3 out]
        n1969 = case shown="False" w4545 {
          tunnel: [w4574 _] -> w4554
          tunnel: w4551 -> [w4573 _]
          frame False {
            w4561 = T11 {"command"="", "command data"=variant} ("element")
            w4560 = "MEAS.mux6_1"
            n1970 = To Variant(anything=T4."mux6-1_channel0" ("mux6_1(3wires)_encode")) -> (Variant=w4559:variant)
            n1971 = To Variant(anything=T4."mux6_1_channel6_3" ("mux6_1(3wires)_encode")) -> (Variant=w4571:variant)
            n1972 = To Variant(anything=T4."mux6_1_channel6_2" ("mux6_1(3wires)_encode")) -> (Variant=w4569:variant)
            n1973 = Bundle By Name(cluster=w4561, "command"=w4560, "command data"=w4569) -> (w4568:T11)
            n1974 = Bundle By Name(cluster=w4561, "command"=w4560, "command data"=w4571) -> (w4567:T11)
            n1975 = Bundle By Name(cluster=w4561, "command"=w4560, "command data"=w4559) -> ()  [unwired: 1 out]
            n1976 = Bundle By Name(cluster=w4561, "command"="MEAS.DMM dual read") -> (w4565:T11)
            n1977 = Build Array(w4568, w4567, w4565) -> (w4563:T11[])
            n1978 = Reverse 1D Array(array=w4563) -> (reversed array=w4564:T11[])
            n1979 = for {
              tunnel: [w4580] -> w4574 mode=indexing
              tunnel: w4573 -> [w4579]
              tunnel: w4564 -> [w4578] mode=indexing
              n1980 = Unbundle By Name(w4578) -> ("command"=w4577:string, "command data"=w4576:variant)
              n1981 = call "App enquece.vi"("Priority Enquece"=TRUE, "command data"=w4576, "command"=w4577, "queue in"=w4579) -> ("error out"=w4580:errorcluster)  [unwired: 6 in, 1 out]
            }
          }
          frame True {
          }
        }
        n1982 = Merge Errors(w4552, w4554) -> (w4553:errorcluster)
      }
      frame "Test DRV 25" {
        w4587 = 25  # DUT index(0-59)
        n1983 = disable-structure shown="LOGGING==TRUE" {
          disable-tunnel: w4588 -> [w4623 _]
          frame condition #0 (active) {
            n1984 = Empty String/Path?(string/path=w4623) -> (empty?=w4626:bool)
            n1985 = Select(t="Quece timeout", s=w4626, f=w4623) -> (s? t:f=w4622:string)
            n1986 = call "string log (SubVI).vi"("Enum"=enum16{"Init", "Log", "Read"}."Log", "state Name"=w4622) -> ()  [unwired: 8 in, 2 out]
          }
          frame condition #1 {
          }
        }
        n1987 = call "progress string(SubVI).vi"("String 3"=w4588, "String in"=w4589) -> ("String out"=w4590:string)  [unwired: 9 in]
        n1988 = call "FGV Driver Data.vi"("DUT index(1-60)"=w4587) -> ("DUT SC"=w4586:bool)  [unwired: 7 in, 3 out]
        n1989 = case shown="False" w4586 {
          tunnel: [w4615 _] -> w4595
          tunnel: w4592 -> [w4614 _]
          frame False {
            w4602 = T11 {"command"="", "command data"=variant} ("element")
            w4601 = "MEAS.mux6_1"
            n1990 = To Variant(anything=T4."mux6-1_channel0" ("mux6_1(3wires)_encode")) -> (Variant=w4600:variant)
            n1991 = To Variant(anything=T4."mux6_1_channel1_3" ("mux6_1(3wires)_encode")) -> (Variant=w4612:variant)
            n1992 = To Variant(anything=T4."mux6-1_channel1_2" ("mux6_1(3wires)_encode")) -> (Variant=w4610:variant)
            n1993 = Bundle By Name(cluster=w4602, "command"=w4601, "command data"=w4610) -> (w4609:T11)
            n1994 = Bundle By Name(cluster=w4602, "command"=w4601, "command data"=w4612) -> (w4608:T11)
            n1995 = Bundle By Name(cluster=w4602, "command"=w4601, "command data"=w4600) -> ()  [unwired: 1 out]
            n1996 = Bundle By Name(cluster=w4602, "command"="MEAS.DMM dual read") -> (w4606:T11)
            n1997 = Build Array(w4609, w4608, w4606) -> (w4604:T11[])
            n1998 = Reverse 1D Array(array=w4604) -> (reversed array=w4605:T11[])
            n1999 = for {
              tunnel: [w4621] -> w4615 mode=indexing
              tunnel: w4614 -> [w4620]
              tunnel: w4605 -> [w4619] mode=indexing
              n2000 = Unbundle By Name(w4619) -> ("command"=w4618:string, "command data"=w4617:variant)
              n2001 = call "App enquece.vi"("Priority Enquece"=TRUE, "command data"=w4617, "command"=w4618, "queue in"=w4620) -> ("error out"=w4621:errorcluster)  [unwired: 6 in, 1 out]
            }
          }
          frame True {
          }
        }
        n2002 = Merge Errors(w4593, w4595) -> (w4594:errorcluster)
      }
      frame "Test DRV 26" {
        w4628 = 26  # DUT index(0-59)
        n2003 = disable-structure shown="LOGGING==TRUE" {
          disable-tunnel: w4629 -> [w4664 _]
          frame condition #0 (active) {
            n2004 = Empty String/Path?(string/path=w4664) -> (empty?=w4667:bool)
            n2005 = Select(t="Quece timeout", s=w4667, f=w4664) -> (s? t:f=w4663:string)
            n2006 = call "string log (SubVI).vi"("Enum"=enum16{"Init", "Log", "Read"}."Log", "state Name"=w4663) -> ()  [unwired: 8 in, 2 out]
          }
          frame condition #1 {
          }
        }
        n2007 = call "progress string(SubVI).vi"("String 3"=w4629, "String in"=w4630) -> ("String out"=w4631:string)  [unwired: 9 in]
        n2008 = call "FGV Driver Data.vi"("DUT index(1-60)"=w4628) -> ("DUT SC"=w4627:bool)  [unwired: 7 in, 3 out]
        n2009 = case shown="False" w4627 {
          tunnel: [w4656 _] -> w4636
          tunnel: w4633 -> [w4655 _]
          frame False {
            w4643 = T11 {"command"="", "command data"=variant} ("element")
            w4642 = "MEAS.mux6_1"
            n2010 = To Variant(anything=T4."mux6-1_channel0" ("mux6_1(3wires)_encode")) -> (Variant=w4641:variant)
            n2011 = To Variant(anything=T4."mux6_1_channel2_3" ("mux6_1(3wires)_encode")) -> (Variant=w4653:variant)
            n2012 = To Variant(anything=T4."mux6_1_channel2_2" ("mux6_1(3wires)_encode")) -> (Variant=w4651:variant)
            n2013 = Bundle By Name(cluster=w4643, "command"=w4642, "command data"=w4651) -> (w4650:T11)
            n2014 = Bundle By Name(cluster=w4643, "command"=w4642, "command data"=w4653) -> (w4649:T11)
            n2015 = Bundle By Name(cluster=w4643, "command"=w4642, "command data"=w4641) -> ()  [unwired: 1 out]
            n2016 = Bundle By Name(cluster=w4643, "command"="MEAS.DMM dual read") -> (w4647:T11)
            n2017 = Build Array(w4650, w4649, w4647) -> (w4645:T11[])
            n2018 = Reverse 1D Array(array=w4645) -> (reversed array=w4646:T11[])
            n2019 = for {
              tunnel: [w4662] -> w4656 mode=indexing
              tunnel: w4655 -> [w4661]
              tunnel: w4646 -> [w4660] mode=indexing
              n2020 = Unbundle By Name(w4660) -> ("command"=w4659:string, "command data"=w4658:variant)
              n2021 = call "App enquece.vi"("Priority Enquece"=TRUE, "command data"=w4658, "command"=w4659, "queue in"=w4661) -> ("error out"=w4662:errorcluster)  [unwired: 6 in, 1 out]
            }
          }
          frame True {
          }
        }
        n2022 = Merge Errors(w4634, w4636) -> (w4635:errorcluster)
      }
